vi "tagDB_SetLock.vi"(8 "error in (no error)":errorcluster, 10 "Lock?":bool, 11 "DB Ref":T1) -> (0 "error out":errorcluster, 3 "DB Ref(dup)":T1)   [LabVIEW 2014, in "TagDB(dev).lvlib"]
doc: "[Covers: REQ_API_Status]"
uses:
  TagDB(dev).lvlib
  tagDB_Def.ctl
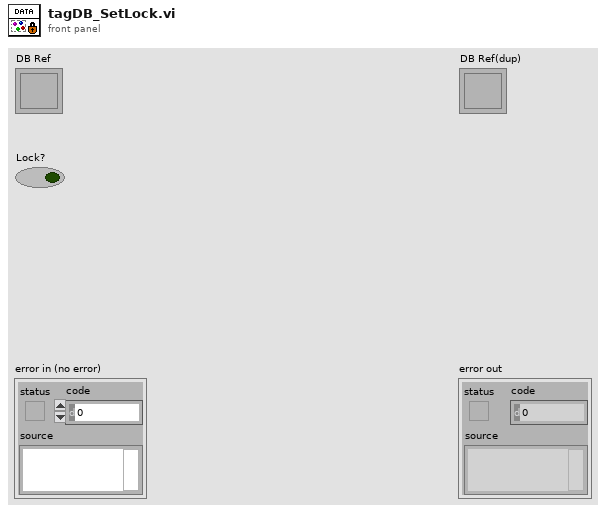
[diagram p1: front panel]
types:
  T1 = typedef "TagDB(dev).lvlib/tagDB_Def.ctl" = refnum<k1>
  T2 = typedef "TagDB(dev).lvlib/_DEF-DATA.ctl" = cluster{"data hashmap":variant, "DataChangeFlag":i64, "ItemChangeFlag":i64, "name":string, "Tag Adding Lock?":bool}
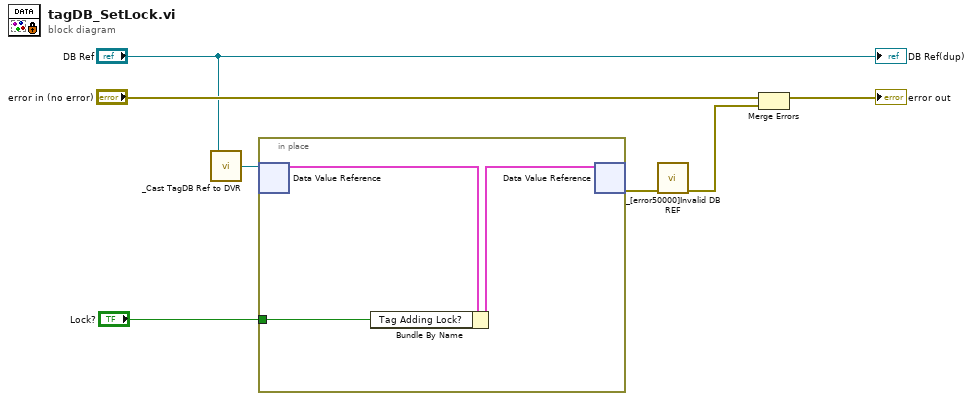
[diagram p0: block diagram]
diagram:
  n1 = call "_Cast TagDB Ref to DVR.vi"("TagDB"="DB Ref") -> ("DVR"=w3:refnum<data-value>)  [unwired: 4 in]
  n2 = in-place {
    in-place-border: "Lock?" -> [w8]
    n3 = in-place-dvr #1(w3) -> (w10:T2)  [unwired: 1 out]
    n4 = Bundle By Name(cluster=w10, "Tag Adding Lock?"=w8) -> (w9:T2)
    n5 = in-place-dvr #1(w9) -> (w2:errorcluster)  [unwired: 1 out]
  }
  n6 = call "_[error50000]Invalid DB REF.vi"("error in (no error)"=w2) -> ("error out"=w1:errorcluster)  [unwired: 10 in]
  n7 = Merge Errors("error in (no error)", w1) -> (→"error out":errorcluster)
  "DB Ref(dup)" <- "DB Ref"
